vi "TextFit_Sort By Order.vi"(8 "Error":errorcluster, 11 "Character Array":T1[](array[typedef])) -> (0 "Error Out":errorcluster, 3 "Character Array Out":T1[](array[typedef]))   [LabVIEW 2014]
doc: "Sorts the character array by order"
uses:
  Controls/Cluster/Cluster_Character Size and Priority Data.ctl
  Controls/String_Picture/String Char Normal.ctl
  Controls/Enum/ENUM_Font Size Select.ctl
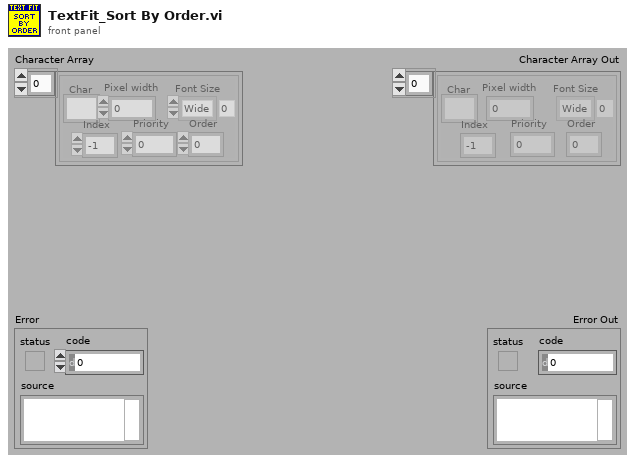
[diagram p1: front panel]
types:
  T1 = typedef "Cluster_Character Size and Priority Data.ctl" = cluster{"Char":T2, "Font Size":T3, "Pixel width":i32, "Priority":i32, "Order":i32, "Index":i32}
  T2 = typedef "String Char Normal.ctl" = string
  T3 = typedef "ENUM_Font Size Select.ctl" = enum16{"Wide", "Med", "Thin"}
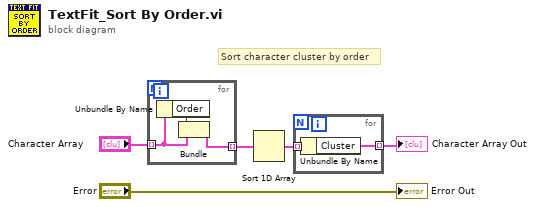
[diagram p0: block diagram]
diagram:
  # "Sort character cluster by order"
  n1 = for {
    tunnel: "Character Array" -> [w7] mode=indexing
    tunnel: [w6] -> w3 mode=indexing
    n2 = Unbundle By Name(w7) -> ("Order"=w8:i32)
    n3 = Bundle("Order"=w8, "Cluster"=w7) -> (w6:cluster{"Order":i32, "Cluster":T1})  [unwired: 1 in]
  }
  n4 = Sort 1D Array(array=w3) -> (sorted array=w4:cluster{"Order":i32, "Cluster":T1}[])
  n5 = for {
    tunnel: w4 -> [w10] mode=indexing
    tunnel: [w9] -> w5 mode=indexing
    n6 = Unbundle By Name(w10) -> ("Cluster"=w9:T1)
  }
  "Character Array Out" <- w5
  "Error Out" <- "Error"
